vi "RF Rec Calculate IQ Power Level.vi"(0 "iq data":cdb[](array[numeric])) -> (4 "power level (dBm)":dbl[](array[numeric]))   [LabVIEW 2018]
doc: "Calculates the power level, in dBm, from the I/Q data."
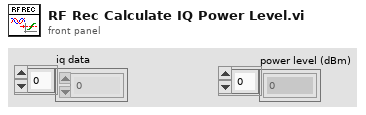
[diagram p1: front panel]
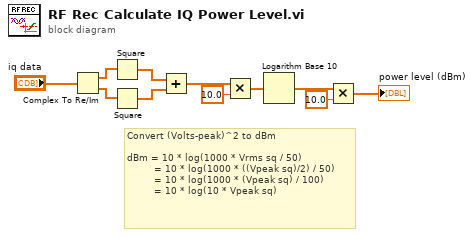
[diagram p0: block diagram]
diagram:
  # "Convert (Volts-peak)^2 to dBm\n\ndBm = 10 * log(1000 * Vrms sq / 50)\n         = 10 * log(1000 * ((Vpeak sq)/2) / 50) \n         = 10 * log(1000 * (Vpeak sq) / 100) \n         = 10 * log(10 * Vpeak sq)"
  n1 = Complex To Re/Im(x + iy="iq data") -> (x=w10:dbl[], y=w9:dbl[])
  n2 = Square(x=w10) -> (x^2=w8:dbl[])
  n3 = Square(x=w9) -> (x^2=w7:dbl[])
  n4 = Add(x=w8, y=w7) -> (x+y=w2:dbl[])
  n5 = Multiply(x=w2, y=10.0) -> (x*y=w4:dbl[])
  n6 = Logarithm Base 10(1:w4) -> (0:w3:dbl[])
  n7 = Multiply(x=w3, y=10.0) -> (x*y=→"power level (dBm)":dbl[])
